vi "test Validate Aliases.vi"(8 "error in (no error)":errorcluster, 11 "TestCase in":refnum<class "Routing and Faulting Validation Unit Tests.lvclass">) -> (0 "error out":errorcluster, 3 "TestCase out":refnum<class "Routing and Faulting Validation Unit Tests.lvclass">)   [LabVIEW 2020, in "Routing and Faulting Validation Unit Tests.lvclass"]
uses:
  Routing and Faulting Validation Unit Tests.lvclass
  Routing and Faulting Validation Unit Tests.lvclass/Routing and Faulting Validation Unit Tests.ctl
  <vilib>/addons/_JKI Toolkits/VI Tester/TestCase.llb/TestCase.lvclass
  Routing and Faulting Scripting.lvlib
  C:/Program Files (x86)/National Instruments/LabVIEW 2020/vi.lib/addons/_JKI Toolkits/VI Tester/TestCase.llb/TestCase.lvclass
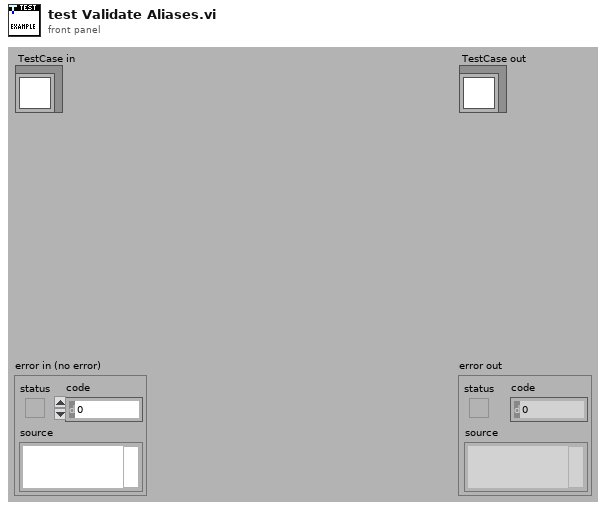
[diagram p1: front panel]
types:
  T1 = typedef "Custom Device API.lvlib/Custom Device Item Ref.ctl" = u64
  T2 = typedef "Routing and Faulting Scripting.lvlib/Validation Information.ctl" = cluster{"Missing Modules":variant, "Module Connection Map":variant, "Unused Modules":variant}
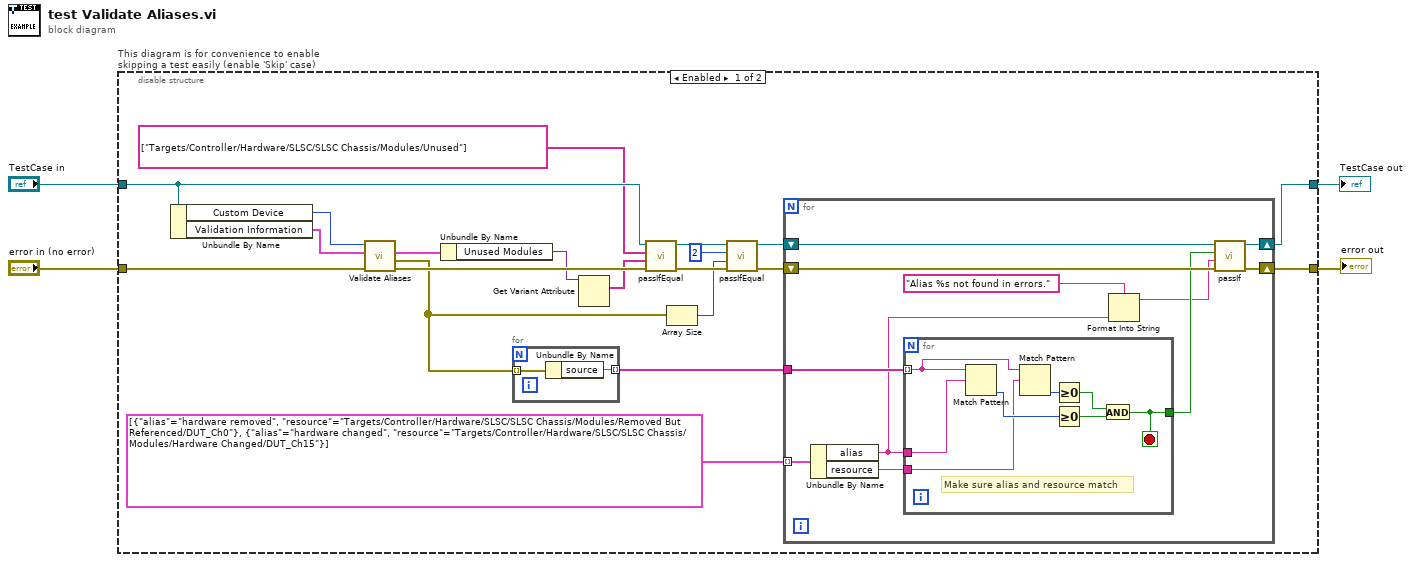
[diagram p0: block diagram]
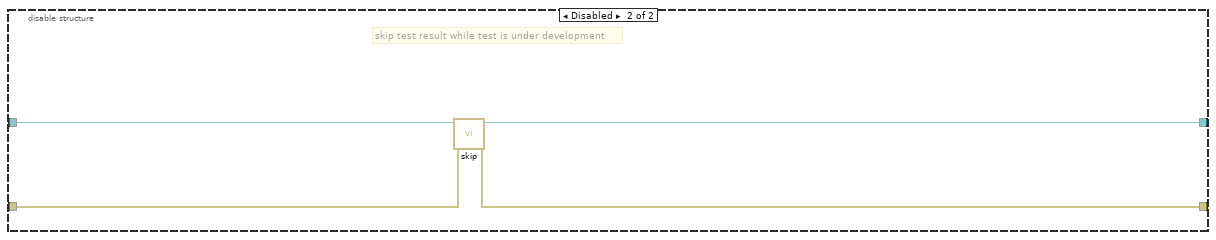
[diagram p2: hidden frame]
diagram:
  n1 = disable-structure "This diagram is for convenience to enable skipping a test easily (enable 'Skip' case)" shown="Enabled" {
    disable-tunnel: "TestCase in" -> [w17 w49]
    disable-tunnel: [w6 w47] -> w1
    disable-tunnel: [w7 w48] -> w3
    disable-tunnel: "error in (no error)" -> [w24 w46]
    frame Enabled {
      n2 = Unbundle By Name(w17) -> ("Custom Device"=w21:T1, "Validation Information"=w22:T2)
      n3 = call "Validate Aliases.vi"("error in"=w24, "validation information in"=w22, "routing and faulting in"=w21) -> ("error out"=w23:errorcluster, "aliases errors"=w10:errorcluster[], "validation information out"=w20:T2)  [unwired: 5 in, 1 out]
      n4 = Unbundle By Name(w20) -> ("Unused Modules"=w19:variant)
      n5 = for {
        tunnel: w10 -> [w26] mode=indexing
        tunnel: [w25] -> w9 mode=indexing
        n6 = Unbundle By Name(w26) -> ("source"=w25:string)
      }
      n7 = Get Variant Attribute(Variant=w19) -> (names=w15:string[])  [unwired: 3 in, 3 out]
      n8 = call-dynamic "passIfEqual.vi"("error in (no error)"=w23, "y"=w15, "x"=string[] ["Targets/Controller/Hardware/SLSC/SLSC Chassis/Modules/Unused"] ("names"), "TestCase in"=w17) -> ("error out"=w18:errorcluster, "TestCase out"=w13:refnum<class "Routing and Faulting Validation Unit Tests.lvclass">)  [unwired: 6 in]
      n9 = Array Size(array=w10) -> (size(s)=w14:i32)
      n10 = call-dynamic "passIfEqual.vi"("error in (no error)"=w18, "y"=w14, "x"=2 ("size(s)"), "TestCase in"=w13) -> ("error out"=w11:errorcluster, "TestCase out"=w8:refnum<class "Routing and Faulting Validation Unit Tests.lvclass">)  [unwired: 6 in]
      n11 = for {
        shift-right: [w34] -> w7
        shift-left: w11 -> [w36]
        tunnel: w9 -> [w37]
        shift-right: [w33] -> w6
        shift-left: w8 -> [w35]
        tunnel: cluster{"alias":string, "resource":string}[] [{"alias"="hardware removed", "resource"="Targets/Controller/Hardware/SLSC/SLSC Chassis/Modules/Removed But Referenced/DUT_Ch0"}, {"alias"="hardware changed", "resource"="Targets/Controller/Hardware/SLSC/SLSC Chassis/Modules/Hardware Changed/DUT_Ch15"}] -> [w30] mode=indexing
        n12 = Unbundle By Name(w30) -> ("alias"=w28:string, "resource"=w29:string)
        n13 = for {
          tunnel: w37 -> [w38] mode=indexing
          tunnel: [w41] -> w32
          tunnel: w28 -> [w40]
          tunnel: w29 -> [w39]
          stop <- w41 stop-if-true
          # "Make sure alias and resource match"
          n14 = Match Pattern(string=w38, regular expression=w40) -> (offset past match=w45:i32)  [unwired: 1 in, 3 out]
          n15 = Match Pattern(string=w38, regular expression=w39) -> (offset past match=w44:i32)  [unwired: 1 in, 3 out]
          n16 = Greater Or Equal To 0?(x=w44) -> (x >= 0?=w43:bool)
          n17 = Greater Or Equal To 0?(x=w45) -> (x >= 0?=w42:bool)
          n18 = And(x=w43, y=w42) -> (x .and. y?=w41:bool)
        }
        n19 = Format Into String(format string="Alias %s not found in errors." ("message (\"\")"), w28) -> (resulting string=w27:string)  [unwired: 2 in, 1 out]
        n20 = call-dynamic "passIf.vi"("error in (no error)"=w36, "message (\"\")"=w27, "pass"=w32, "TestCase in"=w35) -> ("error out"=w34:errorcluster, "TestCase out"=w33:refnum<class "Routing and Faulting Validation Unit Tests.lvclass">)  [unwired: 6 in]
      }
    }
    frame Disabled {
      # "skip test result while test is under development"
      n21 = call <vilib>:"skip.vi"("error in (no error)"=w46, "TestCase in"=w49) -> ("error out"=w48:errorcluster, "TestCase out"=w47:refnum<class "Routing and Faulting Validation Unit Tests.lvclass">)  [unwired: 8 in]
    }
  }
  "error out" <- w3
  "TestCase out" <- w1
